vi "Test Basic Operations 3.vi"() -> ()   [LabVIEW 2014, in "Complex Numbers.lvlib"]
uses:
  Complex Numbers.lvlib
  <vilib>/Aledyne-TSXperts/Arduino Compatible Compiler for LabVIEW/Arduino Compatible Compiler for LabVIEW.lvlib
panel:
  out "error out":errorcluster
  in  "error in (no error)":errorcluster
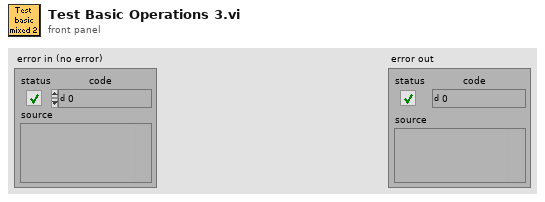
[diagram p1: front panel]
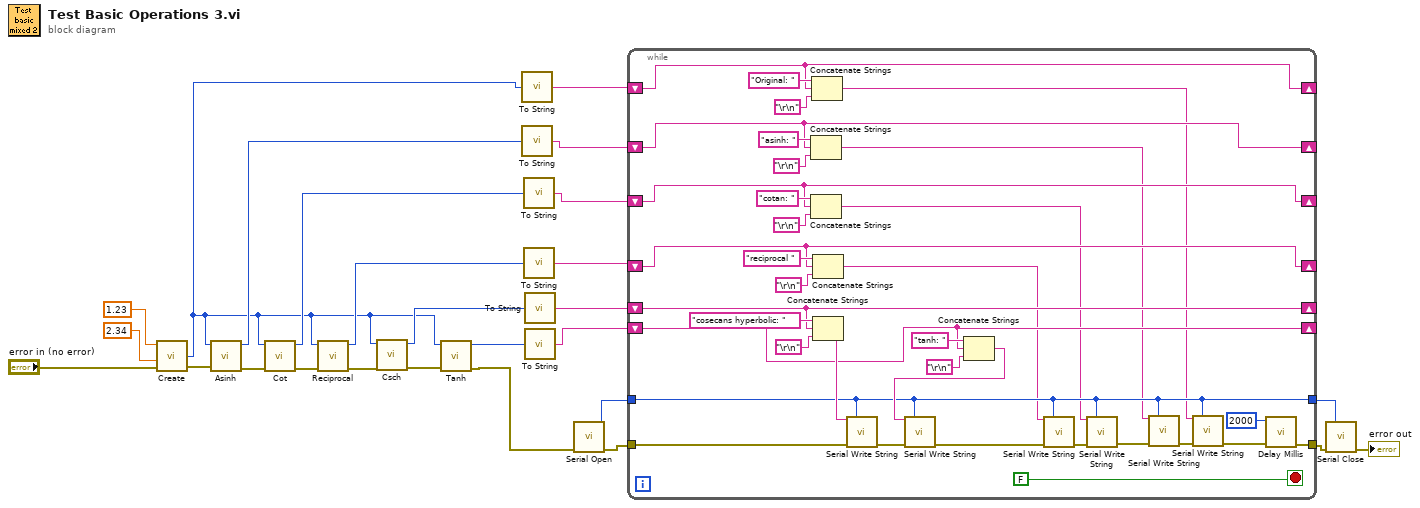
[diagram p0: block diagram]
diagram:
  n1 = call "Create.vi"("Error In"="error in (no error)", "Imag"=2.34, "Real"=1.23) -> ("Error Out"=w12:errorcluster, "Complex"=w1:u32)  [unwired: 2 in]
  n2 = call "Asinh.vi"("Error In"=w12, "A"=w1) -> ("Error Out"=w11:errorcluster, "arcsinh(A)"=w9:u32)  [unwired: 8 in]
  n3 = call "Cot.vi"("Error In"=w11, "A"=w1) -> ("Error Out"=w8:errorcluster, "cotan(A)"=w10:u32)  [unwired: 8 in]
  n4 = call "Reciprocal.vi"("Error In"=w8, "A"=w1) -> ("Error Out"=w7:errorcluster, "reciprocal A"=w5:u32)  [unwired: 8 in]
  n5 = call "Csch.vi"("Error In"=w7, "A"=w1) -> ("Error Out"=w4:errorcluster, "csch(A)"=w6:u32)  [unwired: 8 in]
  n6 = call "Tanh.vi"("Error In"=w4, "A"=w1) -> ("Error Out"=w3:errorcluster, "tanh(A)"=w2:u32)  [unwired: 8 in]
  n7 = call "To String.vi"("Complex number"=w1) -> ("String complex num."=w16:string)
  n8 = call "To String.vi"("Complex number"=w9) -> ("String complex num."=w15:string)
  n9 = call "To String.vi"("Complex number"=w10) -> ("String complex num."=w14:string)
  n10 = call "To String.vi"("Complex number"=w5) -> ("String complex num."=w13:string)
  n11 = call "To String.vi"("Complex number"=w6) -> ("String complex num."=w17:string)
  n12 = call "To String.vi"("Complex number"=w2) -> ("String complex num."=w18:string)
  n13 = call <vilib>:"Serial Open.vi"("error in (no error)"=w3) -> ("Instance"=w24:u8, "error out"=w26:errorcluster)  [unwired: 13 in]
  n14 = while {
    tunnel: w26 -> [w58]
    tunnel: [w60] -> w25
    tunnel: w24 -> [w35]
    tunnel: [w35] -> w23
    shift-right: [w51] -> _
    shift-left: w17 -> [w51]
    shift-right: [w49] -> _
    shift-left: w18 -> [w49]
    shift-right: [w31] -> _
    shift-left: w13 -> [w31]
    shift-right: [w32] -> _
    shift-left: w14 -> [w32]
    shift-right: [w33] -> _
    shift-left: w15 -> [w33]
    shift-right: [w34] -> _
    shift-left: w16 -> [w34]
    stop <- FALSE stop-if-true
    n15 = Concatenate Strings("asinh: " ("string"), w33, "\r\n") -> (w28:string)
    n16 = Concatenate Strings("cotan: " ("string"), w32, "\r\n") -> (w29:string)
    n17 = Concatenate Strings("Original: " ("string"), w34, "\r\n") -> (w27:string)
    n18 = Concatenate Strings("reciprocal " ("string"), w31, "\r\n") -> (w30:string)
    n19 = Concatenate Strings("cosecans hyperbolic: " ("string"), w51, "\r\n") -> (w54:string)
    n20 = call <vilib>:"Serial Write String.vi"("String"=w54, "Instance"=w35, "error in (no error)"=w58) -> ("error out"=w57:errorcluster)  [unwired: 12 in]
    n21 = Concatenate Strings("tanh: " ("string"), w49, "\r\n") -> (w53:string)
    n22 = call <vilib>:"Serial Write String.vi"("String"=w53, "Instance"=w35, "error in (no error)"=w57) -> ("error out"=w37:errorcluster)  [unwired: 12 in]
    n23 = call <vilib>:"Serial Write String.vi"("String"=w30, "Instance"=w35, "error in (no error)"=w37) -> ("error out"=w38:errorcluster)  [unwired: 12 in]
    n24 = call <vilib>:"Serial Write String.vi"("String"=w29, "Instance"=w35, "error in (no error)"=w38) -> ("error out"=w39:errorcluster)  [unwired: 12 in]
    n25 = call <vilib>:"Serial Write String.vi"("String"=w28, "Instance"=w35, "error in (no error)"=w39) -> ("error out"=w40:errorcluster)  [unwired: 12 in]
    n26 = call <vilib>:"Serial Write String.vi"("String"=w27, "Instance"=w35, "error in (no error)"=w40) -> ("error out"=w36:errorcluster)  [unwired: 12 in]
    n27 = call <vilib>:"Delay Millis.vi"("error in (no error)"=w36, "delay"=u32 2000) -> ("error out"=w60:errorcluster)  [unwired: 9 in]
  }
  n28 = call <vilib>:"Serial Close.vi"("Instance"=w23, "error in (no error)"=w25) -> ("error out"=→"error out":errorcluster)  [unwired: 13 in]
